vi "Read Status.vi"(11 "Test Suite Result In":refnum<class "Test Suite Result.lvclass">) -> (2 "Status":T1, 3 "Test Suite Result Out":refnum<class "Test Suite Result.lvclass">)   [LabVIEW 2020, in "Test Suite Result.lvclass"]
uses:
  Test Suite Result.lvclass
  Assertion Result/Public/TypeDefs/Status.ctl
  Test Suite Result.lvclass/Test Suite Result.ctl
  Assertion Result/Assertion Result.lvclass
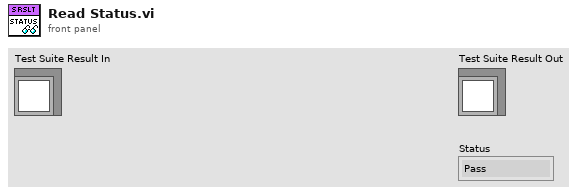
[diagram p1: front panel]
types:
  T1 = typedef "Assertion Result.lvclass/Status.ctl" = enum16{"Pass", "Fail", "Error", "Skipped", "Setup Error", "Broken", "Teardown Error"}
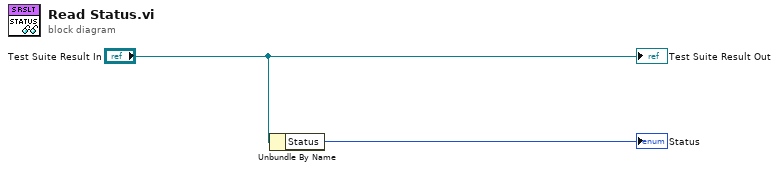
[diagram p0: block diagram]
diagram:
  n1 = Unbundle By Name("Test Suite Result In") -> ("Status"=→"Status":T1)
  "Test Suite Result Out" <- "Test Suite Result In"
